vi "update-frame-data.vi"(8 "error in (no error)":errorcluster, 9 "id":T1 {"payload" format="%x"; "timestamp" format="%<%.7X\n%x>T"; "type" items=["CAN Data"=0, "CAN Remote"=1, "CAN Bus Error"=2, "J1939 Data"=192, "Delay"=224, "Log Trigger"=225, "Start Trigger"=226]; "identifier" format="%x"}, 11 "dbc in":refnum<class "dbc.lvclass">) -> (0 "error out":errorcluster, 1 "CAN frame":T1 {"payload" format="%x"; "timestamp" format="%<%.7X\n%x>T"; "type" items=["CAN Data"=0, "CAN Remote"=1, "CAN Bus Error"=2, "J1939 Data"=192, "Delay"=224, "Log Trigger"=225, "Start Trigger"=226]; "identifier" format="%x"}, 3 "dbc out":refnum<class "dbc.lvclass">)   [LabVIEW 2015, in "dbc.lvclass"]
uses:
  dbc.lvclass
  <vilib>/xnet/xnet.llb/XNET Frame CAN.ctl
  <vilib>/xnet/xnet.llb/XNET Frame Type CAN.ctl
  class.can.table/bAPPdata.lvclass
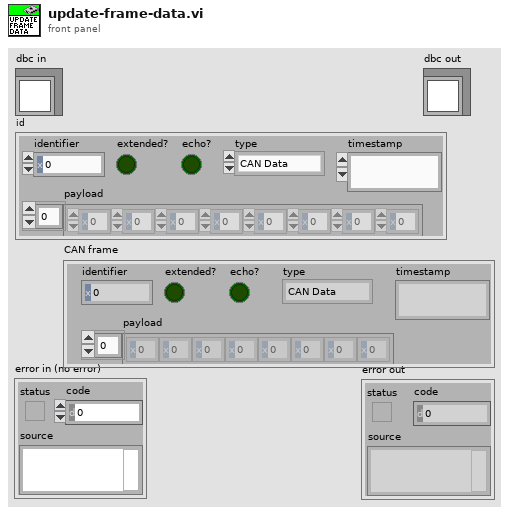
[diagram p1: front panel]
types:
  T1 = typedef "XNET Frame CAN.ctl" = cluster{"timestamp":timestamp, "payload":u8[], "identifier":u32, "type":T2, "extended?":bool, "echo?":bool}
  T2 = typedef "XNET Frame Type CAN.ctl" = u8
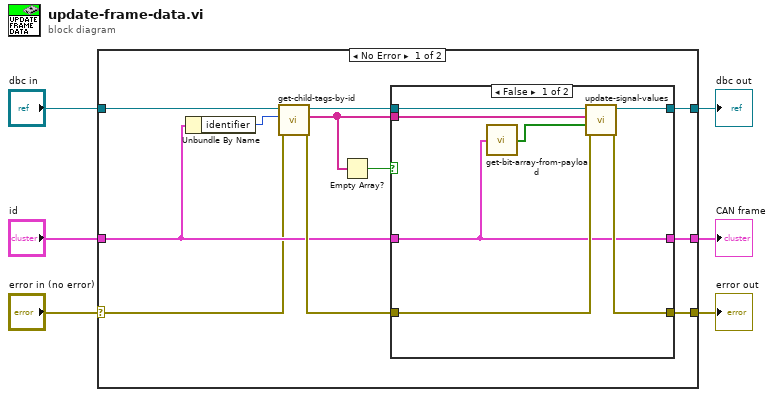
[diagram p0: block diagram]
diagram:
  n1 = case shown="No Error" "error in (no error)" {
    selector: "error in (no error)" -> [w9 w29]
    tunnel: [w16 w29] -> w5
    tunnel: [w14 w28] -> w3
    tunnel: "dbc in" -> [w10 w28]
    tunnel: "id" -> [w11 _]
    tunnel: [w12 _] -> w1
    frame No Error {
      n2 = Unbundle By Name(w11) -> ("identifier"=w7:u32)
      n3 = call "get-child-tags-by-id.vi"("error in (no error)"=w9, "id"=w7, "CANtable in"=w10) -> ("error out"=w15:errorcluster, "child.rags"=w13:string[], "CANtable out"=w17:refnum<class "dbc.lvclass">)  [unwired: 6 in]
      n4 = Empty Array?(array=w13) -> (empty?=w8:bool)
      n5 = case shown="False" w8 {
        tunnel: w17 -> [w20 w27]
        tunnel: [w21 w26] -> w16
        tunnel: w15 -> [w22 w26]
        tunnel: [w24 w27] -> w14
        tunnel: w13 -> [w23 _]
        tunnel: w11 -> [w19 w25]
        tunnel: [w19 w25] -> w12
        frame False {
          n6 = call "get-bit-array-from-payload.vi"("CAN frame"=w19) -> ("Array"=w18:bool[])  [unwired: 4 in]
          n7 = call "update-signal-values.vi"("error in (no error)"=w22, "Array"=w18, "TAGS"=w23, "dbc in"=w20) -> ("error out"=w21:errorcluster, "dbc out"=w24:refnum<class "dbc.lvclass">)  [unwired: 6 in]
        }
        frame True {
        }
      }
    }
    frame Error {
    }
  }
  "error out" <- w5
  "dbc out" <- w3
  "CAN frame" <- w1
